vi "Check Increment Limits.vi"(8 "Increment Limits":dbl[](array[numeric])=[-0.014471871278962644, -0.0027477897622864888, 0.03594582291831433, -0.006177356244415369, -0.000527948512754489, 0.04718526152757189], 9 "Previous":T5, 10 "Current":T5, 11 "Within Limits In":T1) -> (3 "Within Limits Out":T1)   [LabVIEW 2009]
uses:
  Control Loop/Act & Cart Commands.ctl
  Within Limits Matrix.ctl
  Actuator Faults.ctl
  Cart Force Faults.ctl
  Cart Disp Faults.ctl
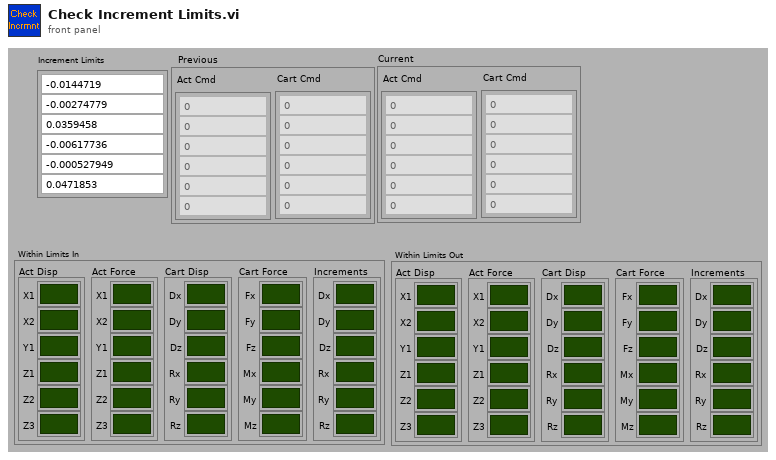
[diagram p1: front panel]
types:
  T1 = typedef "Within Limits Matrix.ctl" = cluster{"Act Disp":T2, "Act Force":T2, "Cart Force":T3, "Cart Disp":T4, "Increments":T4}
  T2 = typedef "Actuator Faults.ctl" = cluster{"X1":bool, "X2":bool, "Y1":bool, "Z1":bool, "Z2":bool, "Z3":bool}
  T3 = typedef "Cart Force Faults.ctl" = cluster{"Fx":bool, "Fy":bool, "Fz":bool, "Mx":bool, "My":bool, "Mz":bool}
  T4 = typedef "Cart Disp Faults.ctl" = cluster{"Dx":bool, "Dy":bool, "Dz":bool, "Rx":bool, "Ry":bool, "Rz":bool}
  T5 = typedef "Act & Cart Commands.ctl" = cluster{"Act Cmd":dbl[], "Cart Cmd":dbl[]}
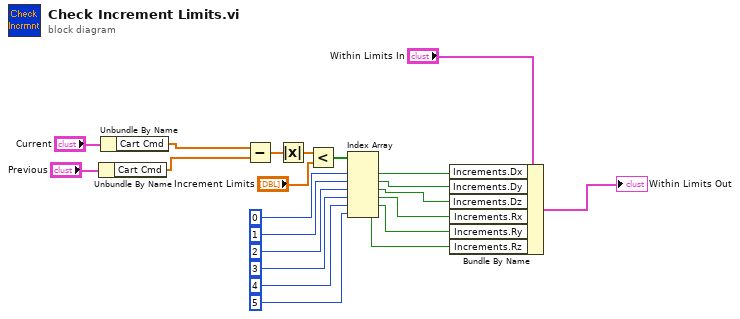
[diagram p0: block diagram]
diagram:
  n1 = Unbundle By Name("Previous") -> ("Cart Cmd"=w19:dbl[])
  n2 = Unbundle By Name("Current") -> ("Cart Cmd"=w20:dbl[])
  n3 = Subtract(x=w20, y=w19) -> (x-y=w18:dbl[])
  n4 = Absolute Value(x=w18) -> (abs(x)=w17:dbl[])
  n5 = Less?(x=w17, y="Increment Limits") -> (x < y?=w13:bool[])
  n6 = Index Array(array=w13, index #1=0 ("index"), index #2=1 ("index"), index #3=2 ("index"), index #4=3 ("index"), index #5=4 ("index"), index #6=5 ("index")) -> (element #1=w6:bool, element #2=w5:bool, element #3=w4:bool, element #4=w3:bool, element #5=w2:bool, element #6=w1:bool)
  n7 = Bundle By Name(cluster="Within Limits In", "Increments.Dx"=w6, "Increments.Dy"=w5, "Increments.Dz"=w4, "Increments.Rx"=w3, "Increments.Ry"=w2, "Increments.Rz"=w1) -> (→"Within Limits Out":T1)
